vi "Get Dependency.vi"(8 "error in (no error)":errorcluster, 11 "Database in":refnum<class "Database.lvclass">) -> (0 "error out":errorcluster, 2 "Dependency":T1, 3 "Database out":refnum<class "Database.lvclass">)   [LabVIEW 2022 SP3, in "Database.lvclass"]
doc: "Developed by Kevin Thompson\nkevin@thompsonengineering.net\n\nCopyright 2018\nThompson Engineering, LLC"
uses:
  Database.lvclass
  DataTypes/Dependency--cluster.ctl
  Database.lvclass/Database.ctl
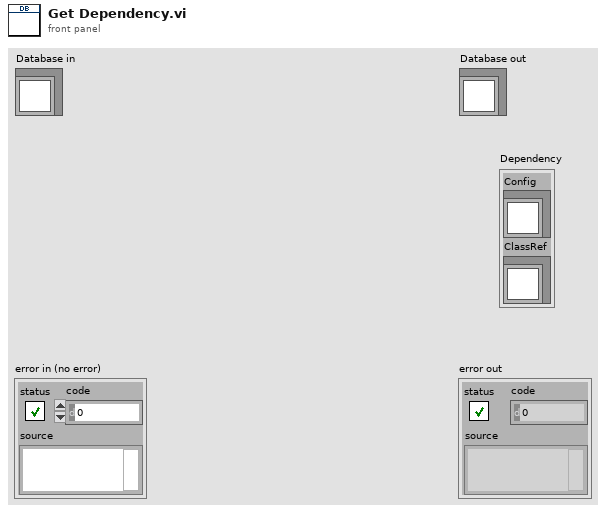
[diagram p1: front panel]
types:
  T1 = typedef "Database.lvclass/Dependency--cluster.ctl" = cluster{"Config":refnum<class>, "ClassRef":refnum<class>}
  T2 = typedef "Database.lvclass/ObjData--cluster.ctl" = cluster{"Settings":T3, "Public Events":T4, "Dependency":T1, "ReadData-placeholder":T5, "VISA-placeholder":refnum<visa-resource-name>}
  T3 = typedef "Database.lvclass/Settings--cluster.ctl" = cluster{"Simulation":bool}
  T4 = typedef "Database.lvclass/Public Events--cluster.ctl" = cluster{"Temp01.AsyncCmd Event":refnum<user-event>, "Temp01.AsyncMsg Event":refnum<user-event>, "stop process":refnum<user-event>, "API Incoming Event":refnum<user-event>, "API Executed Event":refnum<user-event>, "API Return Event":refnum<user-event>}
  T5 = typedef "Database.lvclass/Read Data--cluster.ctl" = cluster{"Data":dbl}
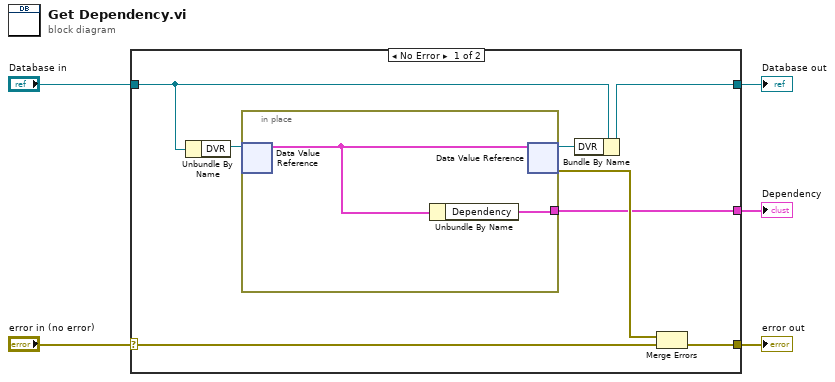
[diagram p0: block diagram]
diagram:
  n1 = case shown="No Error" "error in (no error)" {
    selector: "error in (no error)" -> [w6 w16]
    tunnel: [w7 w16] -> w4
    tunnel: [w9 w17] -> w2
    tunnel: "Database in" -> [w10 w17]
    tunnel: [w8 _] -> w1
    frame No Error {
      n2 = Unbundle By Name(w10) -> ("DVR"=w12:refnum<data-value>)
      n3 = in-place {
        in-place-border: [w14] -> w8
        n4 = in-place-dvr #1(w12) -> (w15:T2)  [unwired: 1 out]
        n5 = Unbundle By Name(w15) -> ("Dependency"=w14:T1)
        n6 = in-place-dvr #1(w15) -> (w13:refnum<data-value>, w11:errorcluster)
      }
      n7 = Bundle By Name(cluster=w10, "DVR"=w13) -> (w9:refnum<class "Database.lvclass">)
      n8 = Merge Errors(w11, w6) -> (w7:errorcluster)
    }
    frame Error {
    }
  }
  "error out" <- w4
  "Database out" <- w2
  "Dependency" <- w1
